vi "Config Get Sections.vi"(8 "error in":errorcluster, 11 "Config Cluster in":T1) -> (0 "error out":errorcluster, 1 "Section Array":string[](array[string]), 3 "Config Cluster out":T1)   [LabVIEW 2017]
uses:
  Config Cluster.ctl
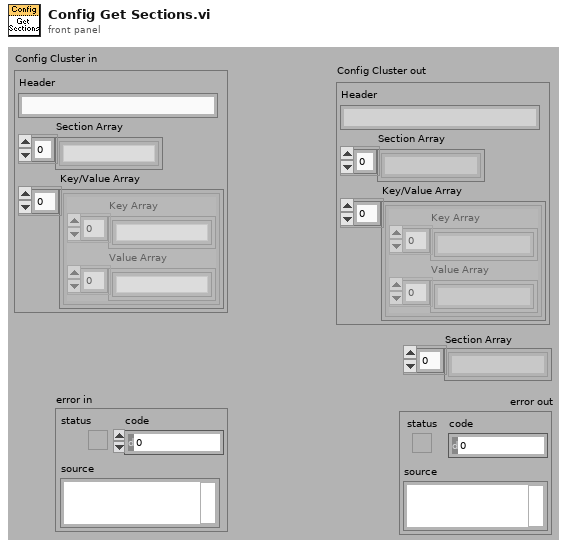
[diagram p1: front panel]
types:
  T1 = typedef "Config Cluster.ctl" = cluster{"Header":string, "Section Array":string[], "Key/Value Array":cluster{"Key Array":string[], "Value Array":string[]}[]}
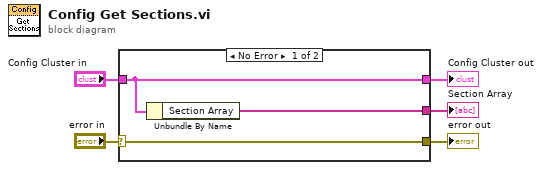
[diagram p0: block diagram]
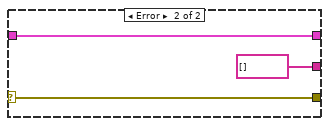
[diagram p2: hidden frame]
diagram:
  n1 = case shown="No Error" "error in" {
    selector: "error in" -> [w8 w11]
    tunnel: "Config Cluster in" -> [w7 w10]
    tunnel: [w8 w11] -> w4
    tunnel: [w7 w10] -> w2
    tunnel: [w6 string[] [] ("Section Array")] -> w1
    frame No Error {
      n2 = Unbundle By Name(w7) -> ("Section Array"=w6:string[])
    }
    frame Error {
    }
  }
  "Config Cluster out" <- w2
  "error out" <- w4
  "Section Array" <- w1
